vi "Set Property Name.vi"(8 "error in":errorcluster, 11 "Property Node in":refnum<k20>) -> (0 "error out":errorcluster, 2 "Property Value":string, 3 "Property Node out":refnum<k20>)   [LabVIEW 2024, in "Config File Parser.lvlib" / "Property.lvclass"]
uses:
  Property.lvclass
  <vilib>/xml/Close Reference(Node).vi
  <resource>/objmgr/DOMUserDefRef.rc
  <vilib>/xml/NI_XML.lvlib
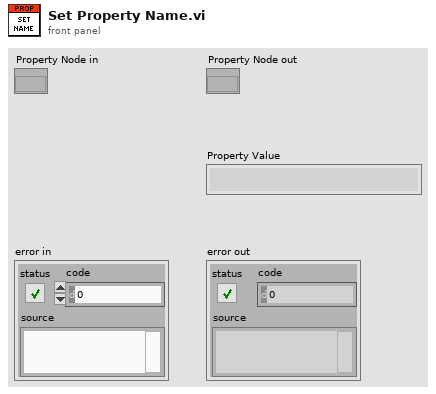
[diagram p1: front panel]
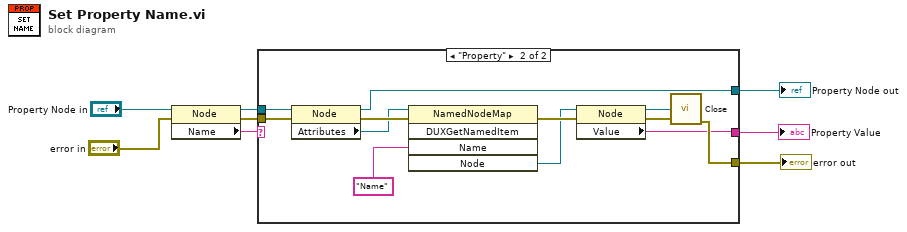
[diagram p0: block diagram]
diagram:
  n1 = property on="Property Node" class="Node"(reference="Property Node in", error in="error in") -> (reference out=w3:refnum<k20>, error out=w6:errorcluster, "Name"=w2:string)
  n2 = case shown="\"Property\"" w2 {
    tunnel: w3 -> [w9 w18]
    tunnel: [_ w16] -> w4
    tunnel: w6 -> [w10 w22]
    tunnel: [w10 w19] -> w8
    tunnel: [w9 w13] -> w1
    frame "-1", Default {
    }
    frame "Property" {
      n3 = property on="Property Node" class="Node"(reference=w18, error in=w22) -> (reference out=w13:refnum<k20>, error out=w21:errorcluster, "Attributes"=w17:refnum<k20>)
      n4 = invoke on="Invoke Node" class="NamedNodeMap" method="DUXGetNamedItem"(reference=w17, error in=w21, "Name"="Name") -> (error out=w20:errorcluster, "Node"=w14:refnum<k20>)  [unwired: 2 in, 3 out]
      n5 = property on="Property Node" class="Node"(reference=w14, error in=w20) -> (reference out=w11:refnum<k20>, error out=w12:errorcluster, "Value"=w16:string)
      n6 = call-poly <vilib>:"Close.vi"("error in (no error)"=w12, "node"=w11) -> ("error out"=w19:errorcluster)  [unwired: 7 in]
    }
  }
  "Property Value" <- w4
  "error out" <- w8
  "Property Node out" <- w1
